vi "LcWebView_AlertDialog_Custom HTML description and buttons with ARIA labels.vi"() -> ()   [LabVIEW 2018, in "LcWebView.lvclass"]
uses:
  LcWebView.lvclass
  webui/ctrls/IconTypeDef.ctl
  C:/Program Files/National Instruments/LabVIEW 2020/user.lib/_LabVIEWCommon/LcWebView/LcWebView_class/data/Microsoft.Web.WebView2.WinForms.dll
panel:
  out "Result":string
  out "BrowserProcessId":u32
  in  "stop":bool
  out "Status Message":string
  in  "Web":refnum<k24>(container)
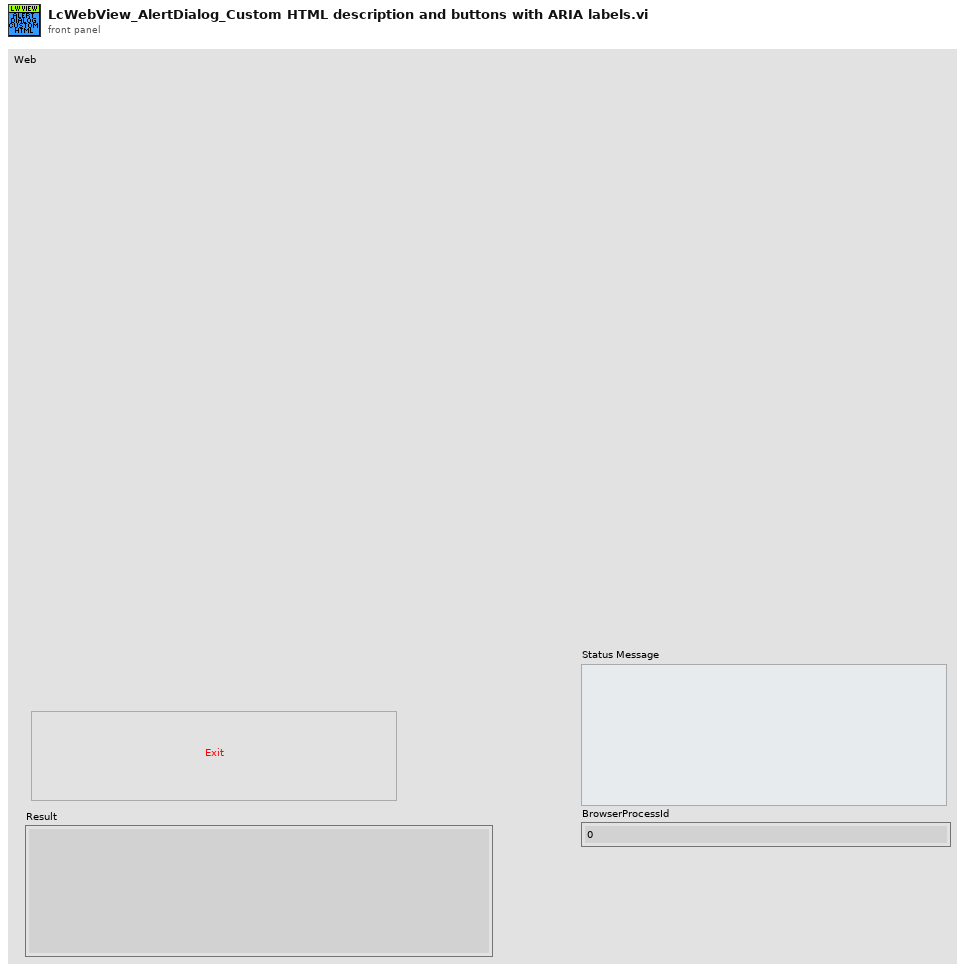
[diagram p1: front panel]
types:
  T1 = typedef "LcWebView.lvclass/IconTypeDef.ctl" = enum16{"success", "error", "warning", "info", "question"}
  T2 = cluster{"title":string, "html":string, "showCloseButton":bool, "showCancelButton":bool, "focusConfirm":bool, "confirmButtonText":string, "confirmButtonAriaLabel":string, "cancelButtonText":string, "cancelButtonAriaLabel":string, "icon":T1}
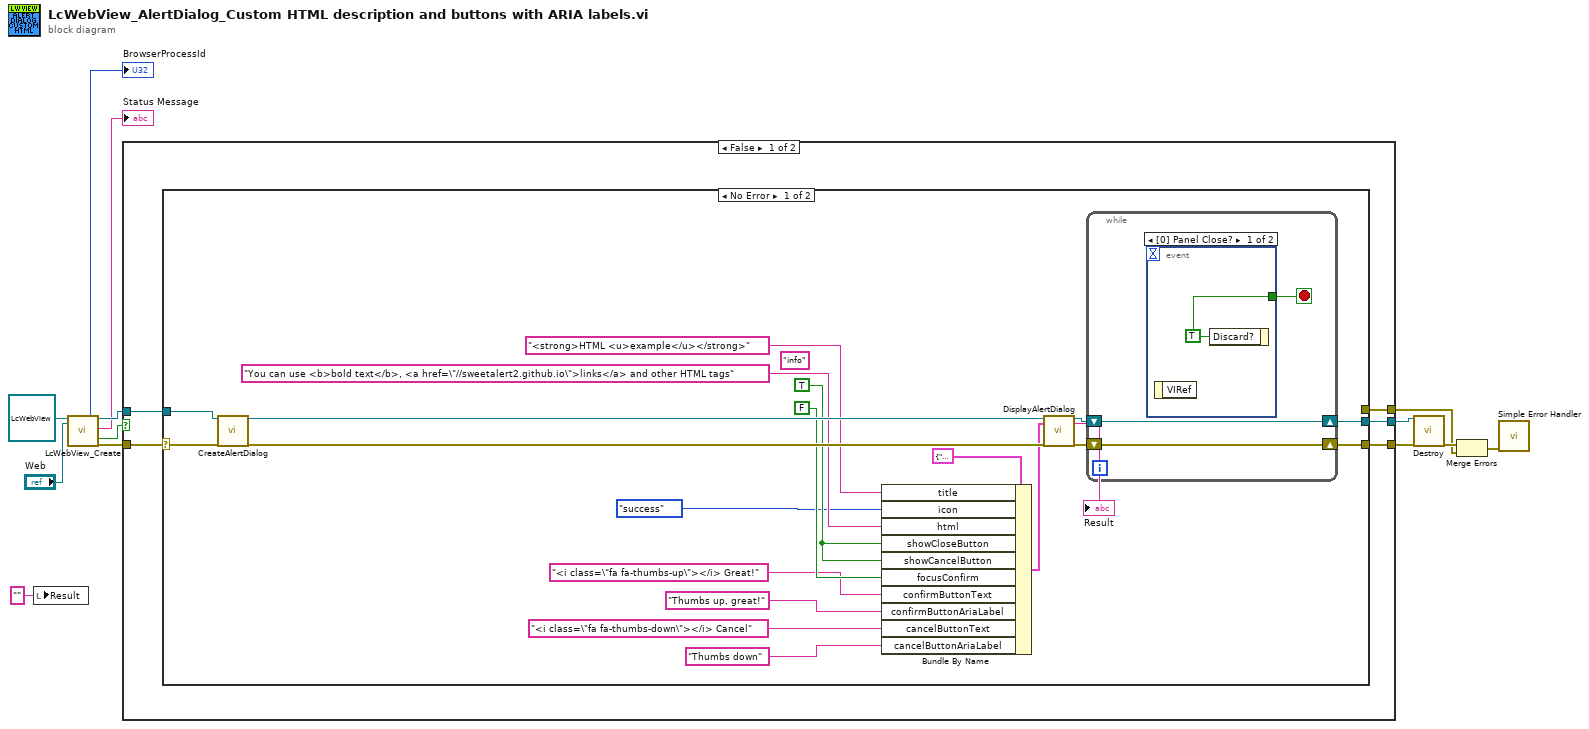
[diagram p0: block diagram]
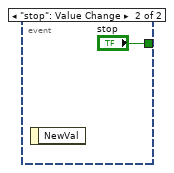
[diagram p2: hidden frame]
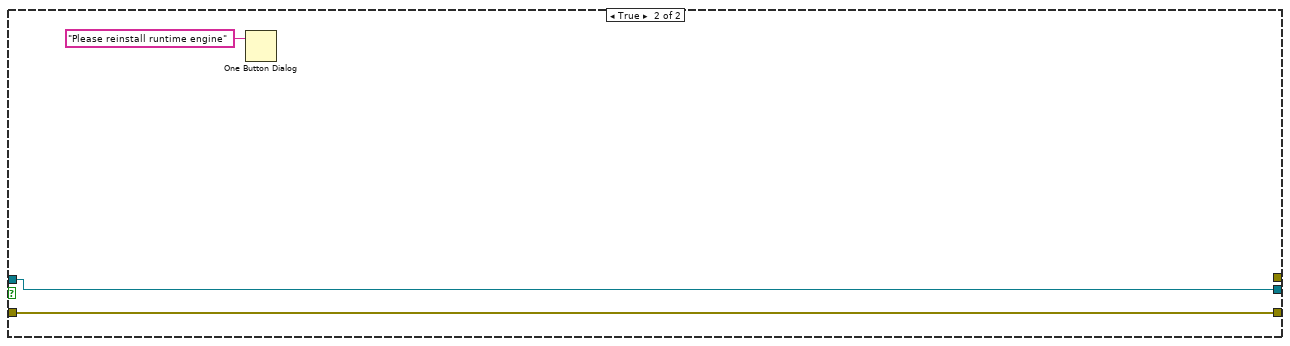
[diagram p4: hidden frame]
diagram:
  n1 = local write "Result"("" ("Result")) -> ()
  n2 = call "LcWebView_Create.vi"("reference in"=refnum<class "LcWebView.lvclass"> refnum, "Webview container"="Web") -> ("BrowserProcessId"=→"BrowserProcessId":u32, "reference out"=w11:refnum<class "LcWebView.lvclass">, "Status Message"=→"Status Message":string, "Reinstall Runtime"=w4:bool, "Error Out"=w10:errorcluster)  [unwired: 10 in, 3 out]
  n3 = case shown="False" w4 {
    tunnel: w11 -> [w18 w48]
    tunnel: w10 -> [w17 w47]
    tunnel: [w16 w48] -> w9
    tunnel: [w14 w47] -> w8
    tunnel: [w15 _] -> w5
    frame False {
      n4 = case shown="No Error" w17 {
        selector: w17 -> [w35 w44]
        tunnel: w18 -> [w36 w45]
        tunnel: [w37 w45] -> w16
        tunnel: [w38 _] -> w14
        tunnel: [_ w44] -> w15
        frame No Error {
          w26 = TRUE ("showCloseButton")
          (unwired) "info" ("text")
          n5 = call-dynamic "CreateAlertDialog.vi"("reference in"=w36, "Error In"=w35) -> ("reference out"=w34:refnum<class "LcWebView.lvclass">, "Error Out"=w33:errorcluster)  [unwired: 16 in]
          n6 = Bundle By Name(cluster=T2 {"title"="", "html"="", "showCloseButton"=FALSE, "showCancelButton"=FALSE, "focusConfirm"=FALSE, "confirmButtonText"="", "confirmButtonAriaLabel"="", "cancelButtonText"="", "cancelButtonAriaLabel"="", "icon"=enum."question"}, "title"="<strong>HTML <u>example</u></strong>", "icon"=IconTypeDef."success", "html"="You can use <b>bold text</b>, <a href=\"//sweetalert2.github.io\">links</a> and other HTML tags", "showCloseButton"=w26, "showCancelButton"=w26, "focusConfirm"=FALSE, "confirmButtonText"="<i class=\"fa fa-thumbs-up\"></i> Great!", "confirmButtonAriaLabel"="Thumbs up, great!", "cancelButtonText"="<i class=\"fa fa-thumbs-down\"></i> Cancel", "cancelButtonAriaLabel"="Thumbs down") -> (w30:T2)
          n7 = call-dynamic "DisplayAlertDialog.vi"("reference in"=w34, "Message"=w30, "Error In"=w33) -> ("reference out"=w32:refnum<class "LcWebView.lvclass">, "Result"=→"Result":string, "Error Out"=w31:errorcluster)  [unwired: 14 in]
          n8 = while {
            shift-right: [w41] -> w37
            shift-left: w32 -> [w41]
            shift-right: [w40] -> w38
            shift-left: w31 -> [w40]
            stop <- w39 stop-if-true
            n9 = event shown="[0] Panel Close?" {
              selector: _ -> [_ _]
              dyn-events: _ -> [_ _]
              timeout: _ -> [_ _]
              tunnel: [w42 "stop"] -> w39
              event Panel Close? {
                w42 = TRUE ("Discard?")
                n10 = event-data() -> ()  [unwired: 1 in, 1 out]
                n11 = event-data("Discard?"=w42) -> ()  [unwired: 1 in, 1 out]
              }
              event "stop": Value Change {
                n12 = event-data() -> ()  [unwired: 1 in, 1 out]
              }
            }
          }
        }
        frame Error {
        }
      }
    }
    frame True {
      n13 = One Button Dialog(message="Please reinstall runtime engine") -> ()  [unwired: 1 in, 1 out]
    }
  }
  n14 = call-dynamic "Destroy.vi"("reference in"=w9, "Error In"=w8) -> ("Error Out"=w7:errorcluster)  [unwired: 16 in, 1 out]
  n15 = Merge Errors(w7, w5) -> (w2:errorcluster)
  n16 = call <vilib>:"Simple Error Handler.vi"("error in (no error)"=w2) -> ()  [unwired: 4 in, 5 out]
